vi "getBounds.vi"(0 "reference":refnum<class "SegmentedLineEdge.lvclass">, 1 "graphics":refnum<class "Graphics.lvclass">, 5 "error in (no error)":errorcluster) -> (14 "reference out":refnum<class "SegmentedLineEdge.lvclass">, 15 "bounds":T1 {"height" format="%.2f"; "width" format="%.2f"; "y" format="%.2f"; "x" format="%.2f"}, 19 "error out":errorcluster)   [LabVIEW 2016, in "SegmentedLineEdge.lvclass"]
doc: "public Rectangle2D getBounds(Graphics2D g2)"
uses:
  <resource>/Framework/Providers/Open_GDS/UML/SegmentedLineEdge_class/SegmentedLineEdge.lvclass
  <resource>/Framework/Providers/Open_GDS/UML/General/Rectangle/Rectangle Rectangle2D.ctl
  <resource>/Framework/Providers/Open_GDS/UML/Graphics_class/Graphics.lvclass
  <resource>/Framework/Providers/Open_GDS/UML/GeneralPathEdge_class/GeneralPathEdge.lvclass
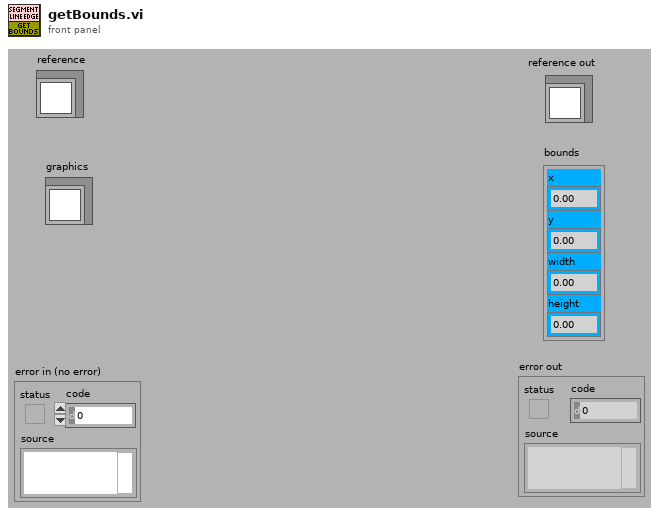
[diagram p1: front panel]
types:
  T1 = typedef "Rectangle Rectangle2D.ctl" = cluster{"x":dbl, "y":dbl, "width":dbl, "height":dbl}
  T2 = typedef "Point Point2D.ctl" = cluster{"x":dbl, "y":dbl}
  T3 = typedef "SegmentedLineEdge.lvclass/ObjectAttributes.ctl" = cluster{"lineStyle":refnum<class "LineStyle.lvclass">, "startArrowHead":refnum<class "ArrowHead.lvclass">, "endArrowHead":refnum<class "ArrowHead.lvclass">, "startLabel":string, "midLabel":string, "endLabel":string, "MidLabelOffset":T2, "SplitWire":bool}
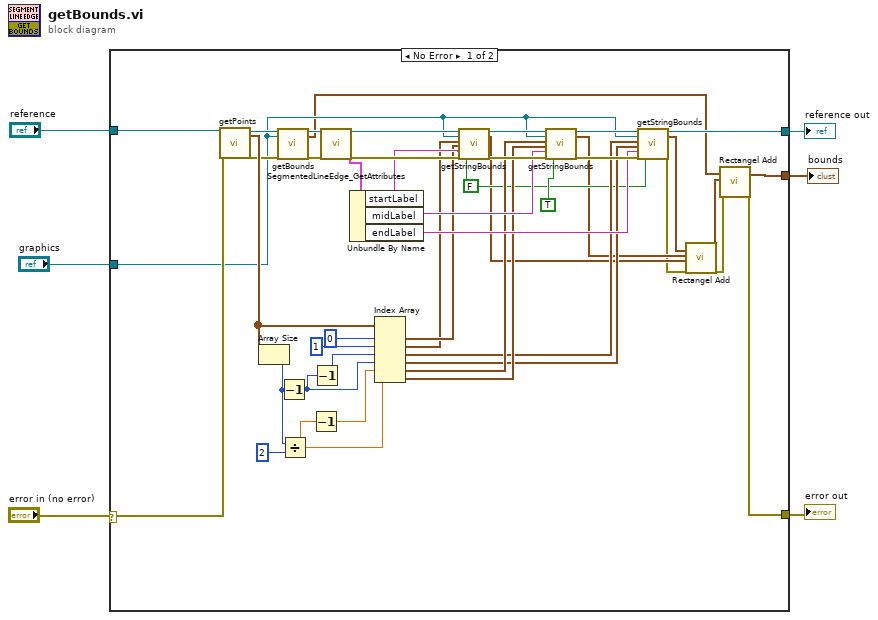
[diagram p0: block diagram]
diagram:
  n1 = case shown="No Error" "error in (no error)" {
    selector: "error in (no error)" -> [w14 w51]
    tunnel: "reference" -> [w50 w52]
    tunnel: [w49 w51] -> w5
    tunnel: [w48 w52] -> w4
    tunnel: "graphics" -> [w9 _]
    tunnel: [w47 _] -> w1
    frame No Error {
      w21 = FALSE ("center")
      n2 = call-dynamic "getPoints.vi"("reference"=w50, "error in (no error)"=w14) -> ("reference out"=w12:refnum<class "SegmentedLineEdge.lvclass">, "points"=w35:T2[], "error out"=w11:errorcluster)  [unwired: 15 in]
      n3 = Array Size(array=w35) -> (size(s)=w29:i32)
      n4 = call-parent "getBounds.vi"("reference"=w12, "graphics"=w9, "error in (no error)"=w11) -> ("reference out"=w13:refnum<class "SegmentedLineEdge.lvclass">, "bounds"=w8:T1, "error out"=w10:errorcluster)  [unwired: 14 in]
      n5 = Decrement(x=w29) -> (x-1=w34:i32)
      n6 = Divide(x=w29, y=2) -> (x/y=w28:dbl)
      n7 = Decrement(x=w28) -> (x-1=w27:dbl)
      n8 = Decrement(x=w34) -> (x-1=w33:i32)
      n9 = call <resource>:"SegmentedLineEdge_GetAttributes.vi"("reference in"=w13, "error in (no error)"=w10) -> ("reference out"=w46:refnum<class "SegmentedLineEdge.lvclass">, "Data"=w7:T3, "error out"=w45:errorcluster)  [unwired: 1 in, 14 out]
      n10 = Unbundle By Name(w7) -> ("startLabel"=w44:string, "midLabel"=w39:string, "endLabel"=w38:string)
      n11 = Index Array(array=w35, index #1=0 ("index"), index #2=1 ("index"), index #3=w33, index #4=w34, index #5=w27, index #6=w28) -> (element #1=w32:T2, element #2=w31:T2, element #3=w24:T2, element #4=w23:T2, element #5=w26:T2, element #6=w25:T2)
      n12 = call-dynamic "getStringBounds.vi"("reference"=w46, "graphics"=w9, "p1"=w31, "p2"=w32, "text"=w44, "error in (no error)"=w45, "center"=w21) -> ("reference out"=w43:refnum<class "SegmentedLineEdge.lvclass">, "bounds"=w20:T1, "error out"=w42:errorcluster)  [unwired: 10 in]
      n13 = call-dynamic "getStringBounds.vi"("reference"=w43, "graphics"=w9, "p1"=w26, "p2"=w25, "text"=w39, "error in (no error)"=w42, "center"=TRUE) -> ("reference out"=w41:refnum<class "SegmentedLineEdge.lvclass">, "bounds"=w19:T1, "error out"=w40:errorcluster)  [unwired: 10 in]
      n14 = call-dynamic "getStringBounds.vi"("reference"=w41, "graphics"=w9, "p1"=w24, "p2"=w23, "text"=w38, "error in (no error)"=w40, "center"=w21) -> ("reference out"=w48:refnum<class "SegmentedLineEdge.lvclass">, "bounds"=w18:T1, "error out"=w16:errorcluster)  [unwired: 10 in]
      n15 = call <resource>:"Rectangel Add.vi"("bounds1"=w18, "bounds2"=w19, "bounds3"=w20, "error in (no error)"=w16) -> ("boundsAdded"=w17:T1, "error out"=w15:errorcluster)  [unwired: 1 in, 13 out]
      n16 = call <resource>:"Rectangel Add.vi"("bounds1"=w8, "bounds2"=w17, "error in (no error)"=w15) -> ("boundsAdded"=w47:T1, "error out"=w49:errorcluster)  [unwired: 2 in, 13 out]
    }
    frame Error {
    }
  }
  "reference out" <- w4
  "error out" <- w5
  "bounds" <- w1
